vi "AutoTask Controller.vi"(8 "error in":errorcluster) -> ()   [LabVIEW 2016]
doc: "This VI executes continuously carrying out the current operation and responding to updates or new operations. It will often contain the timing or control code that is difficult to place directly in TeleOp. This VI generally opens all sensors and motors and isolates the rest of the robot code from knowing how the operations are carried out."
uses:
  AutoTask Setpoints.ctl
  AutoTask Operations.ctl
  <vilib>/Rock Robotics/Network Tables/NT Read Number.vi
  <vilib>/Rock Robotics/Network Tables/NT Write String.vi
  NavX/navX Library v2/navX Library v2.lvlib
  <vilib>/Rock Robotics/Network Tables/NT Write Boolean.vi
panel:
  out "Current\nCmd":string
  # "Tip: It may be helpful to observe inputs and sensor values.\nYou may also want to display tuning or debugging controls."
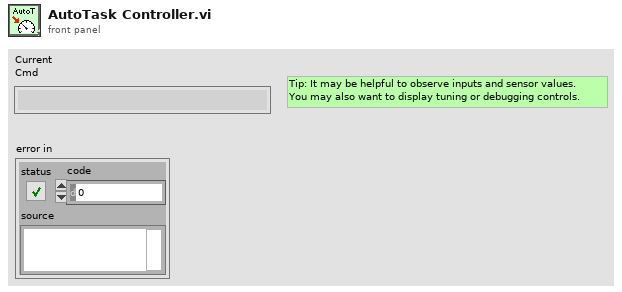
[diagram p1: front panel]
types:
  T1 = typedef "AutoTask Setpoints.ctl" = cluster{"Operation":T2, "Setpoint":dbl, "Duration":dbl, "Speed":dbl, "Angle":dbl, "VDeadband":dbl, "Deadband":dbl}
  T2 = typedef "AutoTask Operations.ctl" = enum16{"Reserve", "Read Current", "Immediate", "DriveDistance", "AutoShoot", "FaceForward", "AutoAlign", "AutoTurn", "DriveToLine", "DriveToIncline", "DriveTillFlat"}
  T3 = typedef "navX Library v2.lvlib/Z900_navX_DeviceTypeDef.ctl" = cluster{"Interface":cluster{"Protocol":T4, "Update Rate (4Hz-60Hz)":u8, "navX Open TypeDef":variant}, "Notify Packet":refnum<notifier>, "Loop VI Refnum":refnum<vi>, "Ready to Close Occurrence Refnum":refnum<k4>}
  T4 = typedef "navX Library v2.lvlib/Z900_navX_ProtocolTypeDef.ctl" = enum16{"SERIAL", "I2C", "SPI"}
  T5 = typedef "Command Status Info.ctl" = cluster{"Name":string, "Status":T6, "notifier out":T7}
  T6 = typedef "Completion Status.ctl" = enum16{"Successful", "Aborted", "Incomplete"}
  T7 = typedef "Completion Notifier.ctl" = refnum<notifier>
  T8 = cluster{"Default Command":T1, "Command Timing":cluster{"Start Time (ms)":u32, "Iterations":i32}, "Command Arguments":cluster{"Command Info":T5, "Description":string, "Default Command":T1, "notifier out":refnum<notifier>, "Subsystem Name":string}}
  T9 = typedef "WPI_EncoderDevRef.ctl" = cluster{"DevStatus":errorcluster, "EncoderIndex":T10, "CounterIndex":T11, "DistancePerCount":dbl, "Decoding Type":T12}
  T10 = typedef "FPGA_EncoderIdx.ctl" = enum8{"Enc 0", "Enc 1", "Enc 2", "Enc 3", "Enc 4", "Enc 5", "Enc 6", "Enc 7", "Invalid"}
  T11 = typedef "FPGA_CounterCtrSystemIndex.ctl" = enum8{"Ctr 0", "Ctr 1", "Ctr 2", "Ctr 3", "Ctr 4", "Ctr 5", "Ctr 6", "Ctr 7", "Invalid"}
  T12 = typedef "WPI_EncoderType.ctl" = enum16{"1x", "2x", "4x"}
  T13 = cluster{"Yaw":dbl, "Roll":dbl, "Pitch":dbl, "Heading":dbl, "Fused Heading":dbl}
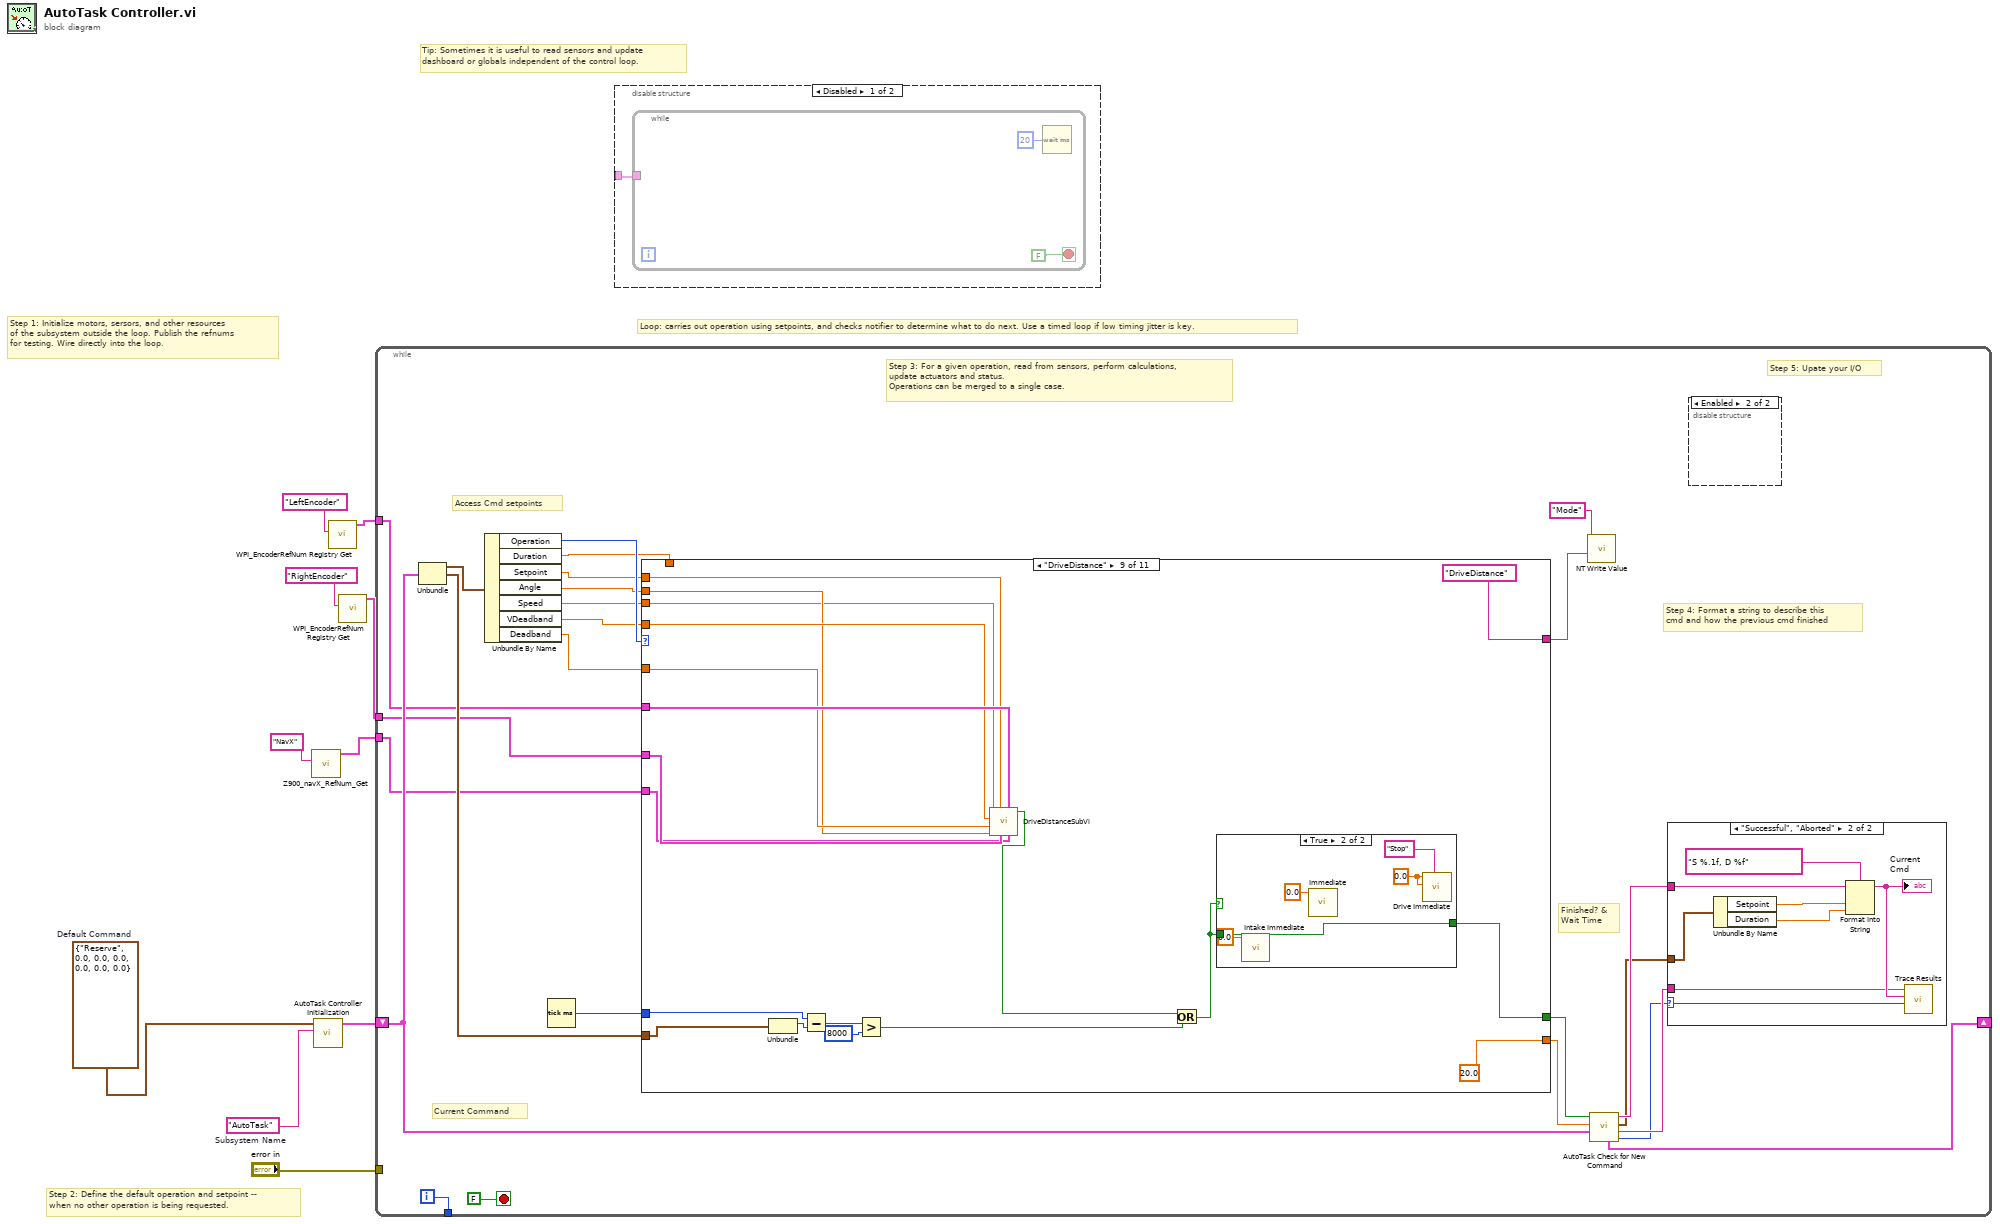
[diagram p0: block diagram]
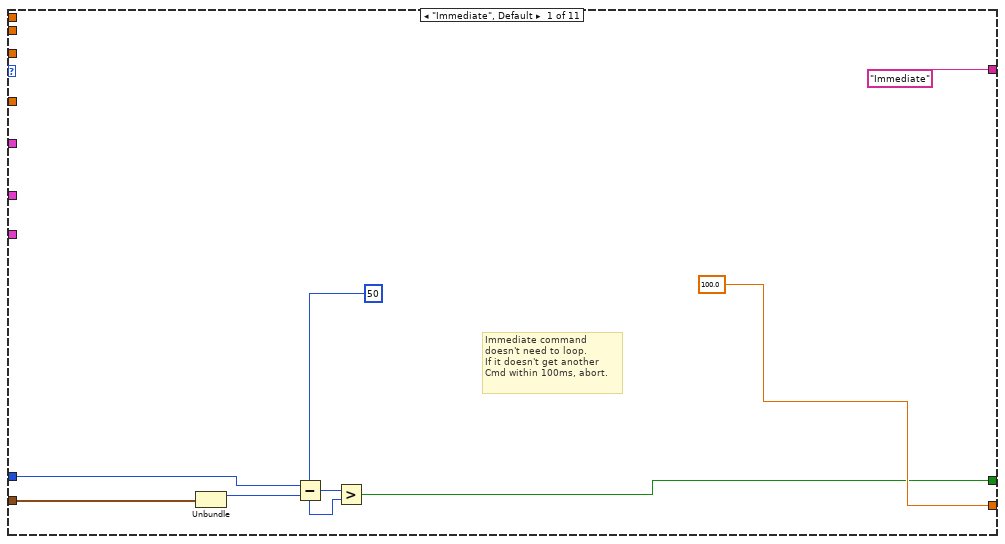
[diagram p3: hidden frame]
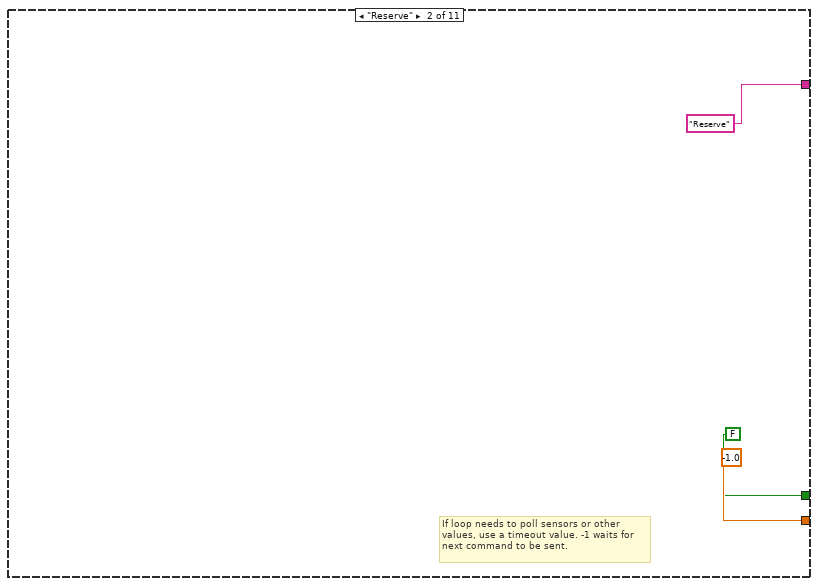
[diagram p4: hidden frame]
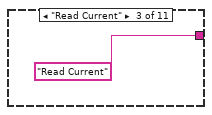
[diagram p5: hidden frame]
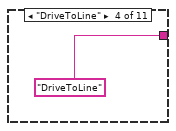
[diagram p6: hidden frame]
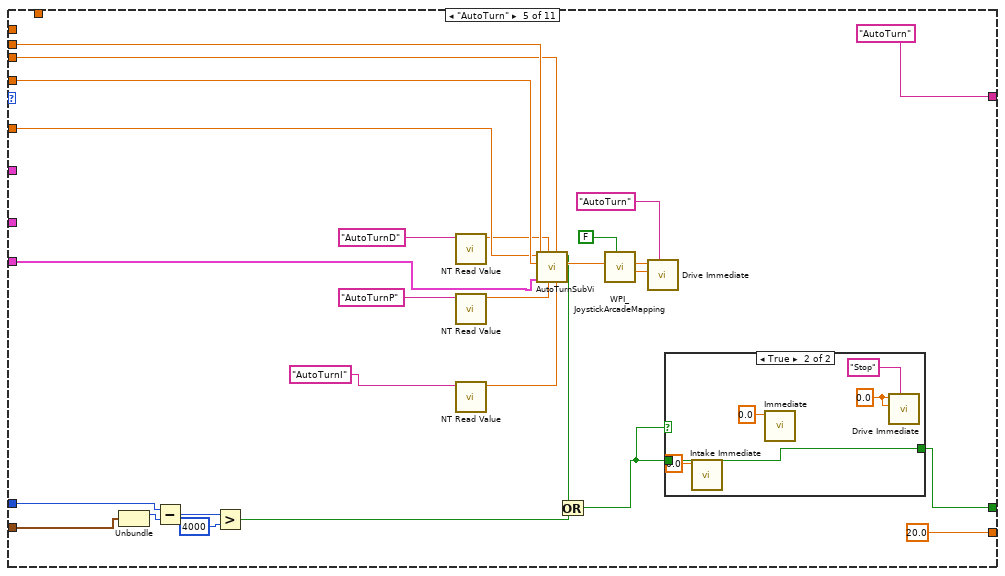
[diagram p7: hidden frame]
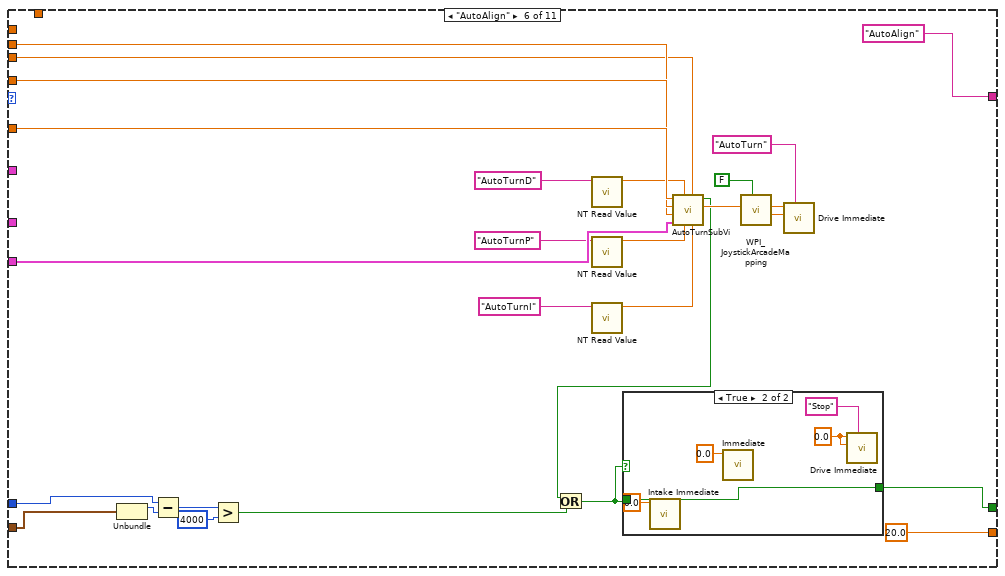
[diagram p9: hidden frame]
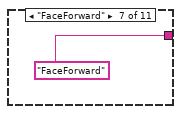
[diagram p11: hidden frame]
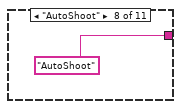
[diagram p12: hidden frame]
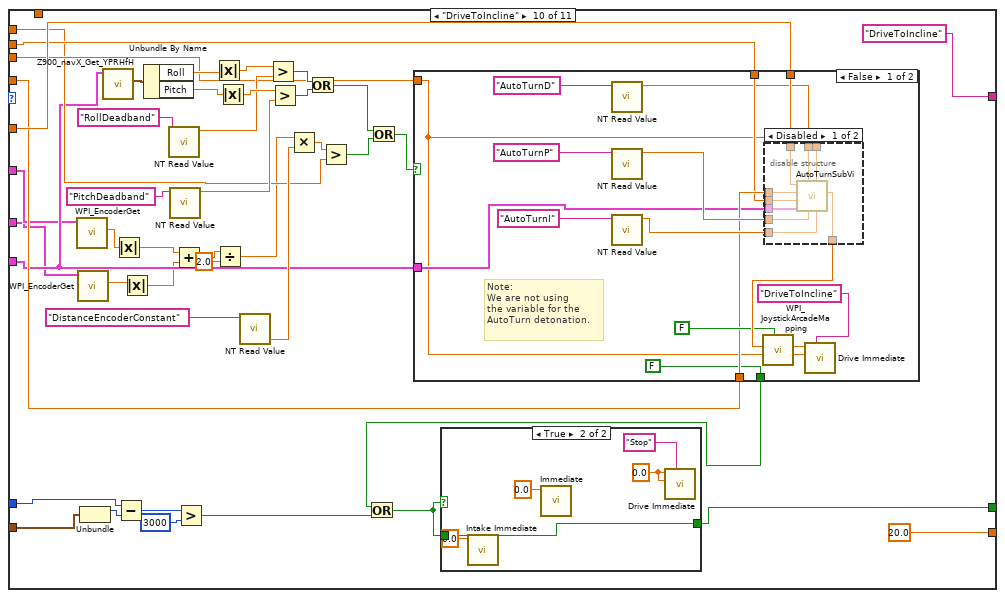
[diagram p14: hidden frame]
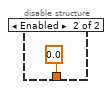
[diagram p16: hidden frame]
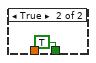
[diagram p17: hidden frame]
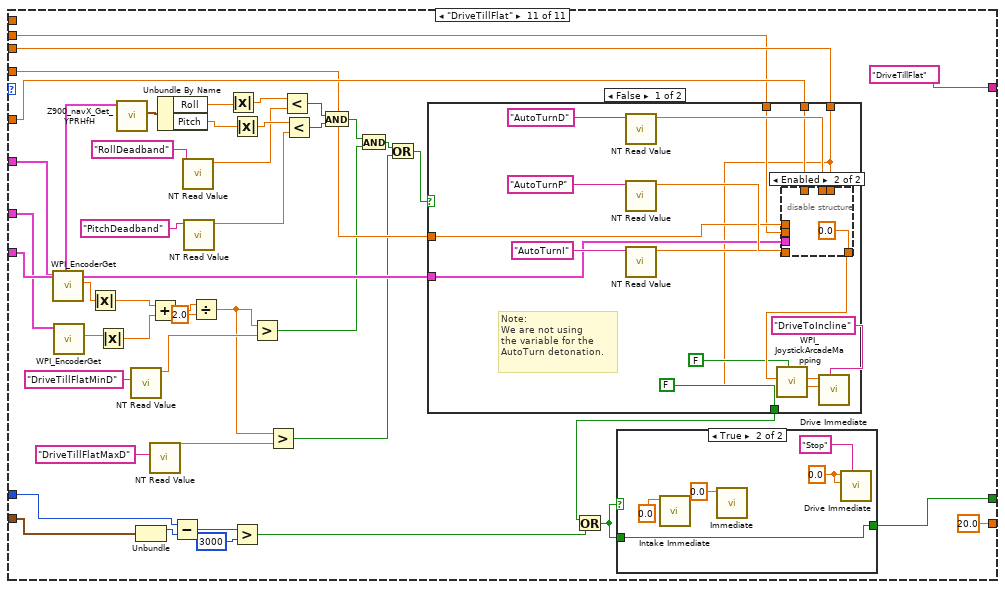
[diagram p18: hidden frame]
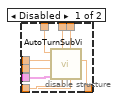
[diagram p20: hidden frame]
diagram:
  w7 = T1 {"Operation"=enum."Reserve", "Setpoint"=0.0, "Duration"=0.0, "Speed"=0.0, "Angle"=0.0, "VDeadband"=0.0, "Deadband"=0.0}  # Default Command
  w8 = "AutoTask"  # Subsystem Name
  # "Tip: Sometimes it is useful to read sensors and update\ndashboard or globals independent of the control loop."
  # "Step 2: Define the default operation and setpoint --\nwhen no other operation is being requested."
  # "Step 1: Initialize motors, sersors, and other resources\nof the subsystem outside the loop. Publish the refnums\nfor testing. Wire directly into the loop."
  # "Loop: carries out operation using setpoints, and checks notifier to determine what to do next. Use a timed loop if low timing jitter is key."
  n1 = call "Z900_navX_RefNum_Get.vi"("refnum name"="NavX") -> ("navX Device"=w6:T3)  [unwired: 9 in, 1 out]
  n2 = call "AutoTask Controller Initialization.vi"("Subsystem Name"=w8, "Default Command"=w7) -> ("Command Info"=w9:T8)  [unwired: 9 in]
  n3 = call <vilib>:"WPI_EncoderRefNum Registry Get.vi"("refnum name"="LeftEncoder") -> ("EncoderDevRef"=w2:T9)  [unwired: 9 in, 1 out]
  n4 = call <vilib>:"WPI_EncoderRefNum Registry Get.vi"("refnum name"="RightEncoder") -> ("EncoderDevRef"=w1:T9)  [unwired: 9 in, 1 out]
  n5 = while {
    shift-right: [w26] -> _
    shift-left: w9 -> [w27]
    tunnel: [w34] -> _
    tunnel: "error in" -> [_]
    tunnel: w6 -> [w19]
    tunnel: w2 -> [w15]
    tunnel: w1 -> [w14]
    i -> [w34]
    stop <- FALSE stop-if-true
    # "Step 5: Upate your I/O"
    # "Step 4: Format a string to describe this\ncmd and how the previous cmd finished"
    # "Current Command"
    # "Access Cmd setpoints"
    # "Finished? &\nWait Time"
    # "Step 3: For a given operation, read from sensors, perform calculations,\nupdate actuators and status.\nOperations can be merged to a single case."
    n6 = Unbundle(w27) -> ("Default Command"=w33:T1, "Command Timing"=w29:cluster{"Start Time (ms)":u32, "Iterations":i32})  [unwired: 1 out]
    n7 = Unbundle By Name(w33) -> ("Operation"=w32:T2, "Duration"=w31:dbl, "Setpoint"=w28:dbl, "Angle"=w18:dbl, "Speed"=w11:dbl, "VDeadband"=w13:dbl, "Deadband"=w12:dbl)
    n8 = Tick Count (ms)() -> (millisecond timer value=w30:u32)
    n9 = case shown="\"DriveDistance\"" w32 {
      tunnel: [100.0 -1.0 _ _ 20.0 20.0 _ _ 20.0 20.0 20.0] -> w24
      tunnel: [w37 FALSE ("ignore previous (F)") _ _ w56 w90 _ _ w125 w150 w227] -> w25
      tunnel: w29 -> [w39 _ _ _ w52 w84 _ _ w119 w144 w221]
      tunnel: w31 -> [_ _ _ _ _ _ _ _ _ _ _]
      tunnel: w30 -> [w38 _ _ _ w51 w85 _ _ w120 w145 w222]
      tunnel: w28 -> [_ _ _ _ _ _ _ _ w132 w164 _]
      tunnel: w19 -> [_ _ _ _ w73 w103 _ _ w126 w160 w247]
      tunnel: w18 -> [_ _ _ _ w74 w105 _ _ w129 w171 w249]
      tunnel: ["Immediate" "Reserve" "Read Current" "DriveToLine" "AutoTurn" "AutoAlign" "FaceForward" "AutoShoot" "DriveDistance" "DriveToIncline" "DriveTillFlat"] -> w16
      tunnel: w13 -> [_ _ _ _ w71 w106 _ _ w131 w172 w250]
      tunnel: w12 -> [_ _ _ _ w70 w107 _ _ w130 w173 w251]
      tunnel: w15 -> [_ _ _ _ _ _ _ _ w134 w159 w237]
      tunnel: w14 -> [_ _ _ _ _ _ _ _ w133 w158 w236]
      tunnel: w11 -> [_ _ _ _ w58 w91 _ _ w127 w170 w252]
      frame "Immediate", Default {
        # "Immediate command\ndoesn't need to loop.\nIf it doesn't get another\nCmd within 100ms, abort."
        n10 = Unbundle(w39) -> ("Start Time (ms)"=w42:u32)  [unwired: 1 out]
        n11 = Subtract(x=w38, y=w42) -> (x-y=w41:u32)
        n12 = Greater?(x=w41, y=u8 50 ("Left Motor")) -> (0:w37:bool)
      }
      frame "Reserve" {
        # "If loop needs to poll sensors or other\nvalues, use a timeout value. -1 waits for\nnext command to be sent."
      }
      frame "Read Current" {
      }
      frame "DriveToLine" {
      }
      frame "AutoTurn" {
        n13 = Unbundle(w52) -> ("Start Time (ms)"=w55:u32)  [unwired: 1 out]
        n14 = Subtract(x=w51, y=w55) -> (x-y=w54:u32)
        n15 = Greater?(x=w54, y=u32 4000 ("Left Motor")) -> (0:w49:bool)
        n16 = call-poly <vilib>:"NT Read Value.vi"("Name"="AutoTurnD") -> ("Numeric"=w60:dbl)  [unwired: 9 in, 1 out]
        n17 = call-poly <vilib>:"NT Read Value.vi"("Name"="AutoTurnP") -> ("Numeric"=w59:dbl)  [unwired: 9 in, 1 out]
        n18 = call-poly <vilib>:"NT Read Value.vi"("Name"="AutoTurnI") -> ("Numeric"=w61:dbl)  [unwired: 9 in, 1 out]
        n19 = call "AutoTurnSubVi.vi"("I"=w61, "Speed"=w58, "P"=w59, "D"=w60, "navX Device"=w73, "Angle"=w74, "VDeadband"=w71, "Deadband"=w70) -> ("Output"=w66:dbl, "Boolean"=w57:bool)  [unwired: 2 in]
        n20 = Or(x=w57, y=w49) -> (x .or. y?=w50:bool)
        n21 = call <vilib>:"WPI_JoystickArcadeMapping.vi"("Square Inputs"=FALSE, "X axis value"=w66) -> ("Right Motor Value"=w68:dbl, "Left Motor Value"=w67:dbl)  [unwired: 8 in]
        n22 = call "Drive Immediate.vi"("Description"="AutoTurn", "Right Setpoint"=w68, "Left Setpoint"=w67) -> ()  [unwired: 8 in, 1 out]
        n23 = case shown="True" w50 {
          tunnel: [w76 w81] -> w56
          tunnel: w50 -> [w76 w81]
          frame False {
          }
          frame True {
            w79 = 0.0
            n24 = call "Intake Immediate.vi"("Setpoint"=0.0) -> ()  [unwired: 10 in, 1 out]
            n25 = call "Immediate.vi"("Setpoint"=0.0) -> ()  [unwired: 10 in, 1 out]
            n26 = call "Drive Immediate.vi"("Description"="Stop", "Right Setpoint"=w79, "Left Setpoint"=w79) -> ()  [unwired: 8 in, 1 out]
          }
        }
      }
      frame "AutoAlign" {
        n27 = Unbundle(w84) -> ("Start Time (ms)"=w89:u32)  [unwired: 1 out]
        n28 = Subtract(x=w85, y=w89) -> (x-y=w88:u32)
        n29 = Greater?(x=w88, y=u32 4000 ("Left Motor")) -> (0:w86:bool)
        n30 = call-poly <vilib>:"NT Read Value.vi"("Name"="AutoTurnD") -> ("Numeric"=w92:dbl)  [unwired: 9 in, 1 out]
        n31 = call-poly <vilib>:"NT Read Value.vi"("Name"="AutoTurnP") -> ("Numeric"=w94:dbl)  [unwired: 9 in, 1 out]
        n32 = call-poly <vilib>:"NT Read Value.vi"("Name"="AutoTurnI") -> ("Numeric"=w93:dbl)  [unwired: 9 in, 1 out]
        n33 = call "AutoTurnSubVi.vi"("I"=w93, "Speed"=w91, "P"=w94, "D"=w92, "navX Device"=w103, "Angle"=w105, "VDeadband"=w106, "Deadband"=w107) -> ("Output"=w98:dbl, "Boolean"=w83:bool)  [unwired: 2 in]
        n34 = Or(x=w83, y=w86) -> (x .or. y?=w82:bool)
        n35 = case shown="True" w82 {
          tunnel: [w109 w114] -> w90
          tunnel: w82 -> [w109 w114]
          frame False {
          }
          frame True {
            w112 = 0.0
            n36 = call "Intake Immediate.vi"("Setpoint"=0.0) -> ()  [unwired: 10 in, 1 out]
            n37 = call "Immediate.vi"("Setpoint"=0.0) -> ()  [unwired: 10 in, 1 out]
            n38 = call "Drive Immediate.vi"("Description"="Stop", "Right Setpoint"=w112, "Left Setpoint"=w112) -> ()  [unwired: 8 in, 1 out]
          }
        }
        n39 = call <vilib>:"WPI_JoystickArcadeMapping.vi"("Square Inputs"=FALSE, "X axis value"=w98) -> ("Right Motor Value"=w101:dbl, "Left Motor Value"=w100:dbl)  [unwired: 8 in]
        n40 = call "Drive Immediate.vi"("Description"="AutoTurn", "Right Setpoint"=w101, "Left Setpoint"=w100) -> ()  [unwired: 8 in, 1 out]
      }
      frame "FaceForward" {
      }
      frame "AutoShoot" {
      }
      frame "DriveDistance" {
        n41 = Unbundle(w119) -> ("Start Time (ms)"=w124:u32)  [unwired: 1 out]
        n42 = Subtract(x=w120, y=w124) -> (x-y=w123:u32)
        n43 = Greater?(x=w123, y=u32 8000 ("Left Motor")) -> (0:w121:bool)
        n44 = call "DriveDistanceSubVi.vi"("navX Device"=w126, "EncoderDevRefLeft"=w134, "EncoderDevRefRight"=w133, "Setpoint"=w132, "Angle"=w129, "Deadband"=w130, "VDeadband"=w131, "Speed"=w127) -> ("Boolean"=w118:bool)  [unwired: 3 in]
        n45 = Or(x=w118, y=w121) -> (x .or. y?=w117:bool)
        n46 = case shown="True" w117 {
          tunnel: [w136 w141] -> w125
          tunnel: w117 -> [w136 w141]
          frame False {
          }
          frame True {
            w139 = 0.0
            n47 = call "Intake Immediate.vi"("Setpoint"=0.0) -> ()  [unwired: 10 in, 1 out]
            n48 = call "Immediate.vi"("Setpoint"=0.0) -> ()  [unwired: 10 in, 1 out]
            n49 = call "Drive Immediate.vi"("Description"="Stop", "Right Setpoint"=w139, "Left Setpoint"=w139) -> ()  [unwired: 8 in, 1 out]
          }
        }
      }
      frame "DriveToIncline" {
        n50 = call <vilib>:"WPI_EncoderGet.vi"("EncoderDevRef"=w159) -> ("Distance"=w156:dbl)  [unwired: 5 in, 5 out]
        n51 = call <vilib>:"WPI_EncoderGet.vi"("EncoderDevRef"=w158) -> ("Distance"=w157:dbl)  [unwired: 5 in, 5 out]
        n52 = Unbundle(w144) -> ("Start Time (ms)"=w149:u32)  [unwired: 1 out]
        n53 = call "Z900_navX_Get_YPRHfH.vi"("navX Device"=w160) -> ("YRPHfH"=w184:T13)  [unwired: 7 in, 3 out]
        n54 = Absolute Value(x=w156) -> (abs(x)=w155:dbl)
        n55 = Subtract(x=w145, y=w149) -> (x-y=w148:u32)
        n56 = Absolute Value(x=w157) -> (abs(x)=w154:dbl)
        n57 = Unbundle By Name(w184) -> ("Roll"=w183:dbl, "Pitch"=w180:dbl)
        n58 = call-poly <vilib>:"NT Read Value.vi"("Name"="RollDeadband") -> ("Numeric"=w177:dbl)  [unwired: 9 in, 1 out]
        n59 = call-poly <vilib>:"NT Read Value.vi"("Name"="PitchDeadband") -> ("Numeric"=w176:dbl)  [unwired: 9 in, 1 out]
        n60 = Add(x=w155, y=w154) -> (x+y=w153:dbl)
        n61 = Greater?(x=w148, y=u32 3000 ("Left Motor")) -> (0:w146:bool)
        n62 = Absolute Value(x=w183) -> (abs(x)=w182:dbl)
        n63 = Divide(x=w153, y=2.0) -> (x/y=w151:dbl)
        n64 = Absolute Value(x=w180) -> (abs(x)=w181:dbl)
        n65 = call-poly <vilib>:"NT Read Value.vi"("Name"="DistanceEncoderConstant") -> ("Numeric"=w166:dbl)  [unwired: 9 in, 1 out]
        n66 = Greater?(x=w182, y=w177) -> (0:w174:bool)
        n67 = Greater?(x=w181, y=w176) -> (0:w175:bool)
        n68 = Multiply(x=w151, y=w166) -> (x*y=w165:dbl)
        n69 = Or(x=w174, y=w175) -> (x .or. y?=w163:bool)
        n70 = Greater?(x=w165, y=w164) -> (0:w162:bool)
        n71 = Or(x=w163, y=w162) -> (x .or. y?=w161:bool)
        n72 = case shown="False" w161 {
          tunnel: w173 -> [w197 _]
          tunnel: w172 -> [w196 _]
          tunnel: w171 -> [w195 _]
          tunnel: w170 -> [w193 _]
          tunnel: w160 -> [w194 _]
          tunnel: [FALSE TRUE] -> w143
          frame False {
            # "Note:\nWe are not using\nthe variable for the\nAutoTurn detonation."
            n73 = call-poly <vilib>:"NT Read Value.vi"("Name"="AutoTurnD") -> ("Numeric"=w191:dbl)  [unwired: 9 in, 1 out]
            n74 = call-poly <vilib>:"NT Read Value.vi"("Name"="AutoTurnP") -> ("Numeric"=w206:dbl)  [unwired: 9 in, 1 out]
            n75 = call-poly <vilib>:"NT Read Value.vi"("Name"="AutoTurnI") -> ("Numeric"=w205:dbl)  [unwired: 9 in, 1 out]
            n76 = disable-structure shown="Disabled" {
              disable-tunnel: [w216 0.0 ("X axis value")] -> w207
              disable-tunnel: w206 -> [w215 _]
              disable-tunnel: w205 -> [w214 _]
              disable-tunnel: w197 -> [w213 _]
              disable-tunnel: w196 -> [w212 _]
              disable-tunnel: w195 -> [w211 _]
              disable-tunnel: w194 -> [w210 _]
              disable-tunnel: w193 -> [w209 _]
              disable-tunnel: w191 -> [w208 _]
              frame Disabled {
                n77 = call "AutoTurnSubVi.vi"("I"=w214, "Speed"=w209, "P"=w215, "D"=w208, "navX Device"=w210, "Angle"=w211, "VDeadband"=w212, "Deadband"=w213) -> ("Output"=w216:dbl)  [unwired: 2 in, 1 out]
              }
              frame Enabled {
              }
            }
            n78 = call <vilib>:"WPI_JoystickArcadeMapping.vi"("Square Inputs"=FALSE, "Y axis value"=w193, "X axis value"=w207) -> ("Right Motor Value"=w199:dbl, "Left Motor Value"=w198:dbl)  [unwired: 7 in]
            n79 = call "Drive Immediate.vi"("Description"="DriveToIncline", "Right Setpoint"=w199, "Left Setpoint"=w198) -> ()  [unwired: 8 in, 1 out]
          }
          frame True {
          }
        }
        n80 = Or(x=w143, y=w146) -> (x .or. y?=w142:bool)
        n81 = case shown="True" w142 {
          tunnel: [w185 w190] -> w150
          tunnel: w142 -> [w185 w190]
          frame False {
          }
          frame True {
            w188 = 0.0
            n82 = call "Intake Immediate.vi"("Setpoint"=0.0) -> ()  [unwired: 10 in, 1 out]
            n83 = call "Immediate.vi"("Setpoint"=0.0) -> ()  [unwired: 10 in, 1 out]
            n84 = call "Drive Immediate.vi"("Description"="Stop", "Right Setpoint"=w188, "Left Setpoint"=w188) -> ()  [unwired: 8 in, 1 out]
          }
        }
      }
      frame "DriveTillFlat" {
        n85 = call <vilib>:"WPI_EncoderGet.vi"("EncoderDevRef"=w237) -> ("Distance"=w238:dbl)  [unwired: 5 in, 5 out]
        n86 = call <vilib>:"WPI_EncoderGet.vi"("EncoderDevRef"=w236) -> ("Distance"=w243:dbl)  [unwired: 5 in, 5 out]
        n87 = Absolute Value(x=w238) -> (abs(x)=w242:dbl)
        n88 = Absolute Value(x=w243) -> (abs(x)=w241:dbl)
        n89 = call "Z900_navX_Get_YPRHfH.vi"("navX Device"=w247) -> ("YRPHfH"=w263:T13)  [unwired: 7 in, 3 out]
        n90 = call-poly <vilib>:"NT Read Value.vi"("Name"="DriveTillFlatMinD") -> ("Numeric"=w233:dbl)  [unwired: 9 in, 1 out]
        n91 = Unbundle(w221) -> ("Start Time (ms)"=w226:u32)  [unwired: 1 out]
        n92 = Add(x=w242, y=w241) -> (x+y=w240:dbl)
        n93 = call-poly <vilib>:"NT Read Value.vi"("Name"="DriveTillFlatMaxD") -> ("Numeric"=w231:dbl)  [unwired: 9 in, 1 out]
        n94 = Unbundle By Name(w263) -> ("Roll"=w262:dbl, "Pitch"=w259:dbl)
        n95 = Subtract(x=w222, y=w226) -> (x-y=w225:u32)
        n96 = call-poly <vilib>:"NT Read Value.vi"("Name"="RollDeadband") -> ("Numeric"=w256:dbl)  [unwired: 9 in, 1 out]
        n97 = call-poly <vilib>:"NT Read Value.vi"("Name"="PitchDeadband") -> ("Numeric"=w255:dbl)  [unwired: 9 in, 1 out]
        n98 = Divide(x=w240, y=2.0) -> (x/y=w230:dbl)
        n99 = Absolute Value(x=w262) -> (abs(x)=w261:dbl)
        n100 = Absolute Value(x=w259) -> (abs(x)=w260:dbl)
        n101 = Greater?(x=w225, y=u32 3000 ("Left Motor")) -> (0:w223:bool)
        n102 = Greater?(x=w230, y=w233) -> (0:w232:bool)
        n103 = Greater?(x=w230, y=w231) -> (0:w229:bool)
        n104 = Less?(x=w261, y=w256) -> (x < y?=w253:bool)
        n105 = Less?(x=w260, y=w255) -> (x < y?=w254:bool)
        n106 = And(x=w253, y=w254) -> (x .and. y?=w246:bool)
        n107 = And(x=w246, y=w232) -> (x .and. y?=w245:bool)
        n108 = Or(x=w245, y=w229) -> (x .or. y?=w244:bool)
        n109 = case shown="False" w244 {
          tunnel: [FALSE TRUE] -> w220
          tunnel: w252 -> [w270 _]
          tunnel: w251 -> [w275 _]
          tunnel: w250 -> [w274 _]
          tunnel: w249 -> [w273 _]
          tunnel: w247 -> [w271 _]
          frame False {
            # "Note:\nWe are not using\nthe variable for the\nAutoTurn detonation."
            n110 = call-poly <vilib>:"NT Read Value.vi"("Name"="AutoTurnD") -> ("Numeric"=w276:dbl)  [unwired: 9 in, 1 out]
            n111 = call-poly <vilib>:"NT Read Value.vi"("Name"="AutoTurnP") -> ("Numeric"=w285:dbl)  [unwired: 9 in, 1 out]
            n112 = call-poly <vilib>:"NT Read Value.vi"("Name"="AutoTurnI") -> ("Numeric"=w272:dbl)  [unwired: 9 in, 1 out]
            n113 = disable-structure shown="Enabled" {
              disable-tunnel: [w295 0.0 ("X axis value")] -> w286
              disable-tunnel: w285 -> [w294 _]
              disable-tunnel: w276 -> [w293 _]
              disable-tunnel: w270 -> [w292 _]
              disable-tunnel: w275 -> [w291 _]
              disable-tunnel: w274 -> [w290 _]
              disable-tunnel: w273 -> [w289 _]
              disable-tunnel: w272 -> [w288 _]
              disable-tunnel: w271 -> [w287 _]
              frame Disabled {
                n114 = call "AutoTurnSubVi.vi"("I"=w288, "Speed"=w292, "P"=w294, "D"=w293, "navX Device"=w287, "Angle"=w289, "VDeadband"=w290, "Deadband"=w291) -> ("Output"=w295:dbl)  [unwired: 2 in, 1 out]
              }
              frame Enabled {
              }
            }
            n115 = call <vilib>:"WPI_JoystickArcadeMapping.vi"("Square Inputs"=FALSE, "Y axis value"=w270, "X axis value"=w286) -> ("Right Motor Value"=w279:dbl, "Left Motor Value"=w278:dbl)  [unwired: 7 in]
            n116 = call "Drive Immediate.vi"("Description"="DriveToIncline", "Right Setpoint"=w279, "Left Setpoint"=w278) -> ()  [unwired: 8 in, 1 out]
          }
          frame True {
          }
        }
        n117 = Or(x=w220, y=w223) -> (x .or. y?=w219:bool)
        n118 = case shown="True" w219 {
          tunnel: [w264 w265] -> w227
          tunnel: w219 -> [w264 w265]
          frame False {
          }
          frame True {
            w268 = 0.0
            n119 = call "Intake Immediate.vi"("Setpoint"=0.0) -> ()  [unwired: 10 in, 1 out]
            n120 = call "Immediate.vi"("Setpoint"=0.0) -> ()  [unwired: 10 in, 1 out]
            n121 = call "Drive Immediate.vi"("Description"="Stop", "Right Setpoint"=w268, "Left Setpoint"=w268) -> ()  [unwired: 8 in, 1 out]
          }
        }
      }
    }
    n122 = call-poly <vilib>:"NT Write Value.vi"("String"=w16, "Name"="Mode") -> ()  [unwired: 9 in, 1 out]
    n123 = call "AutoTask Check for New Command.vi"("Current Command"=w27, "Wait time (ms)"=w24, "Finished?"=w25) -> ("Completion"=w20:T6, "Subsystem Name"=w21:string, "Current Command"=w22:T1, "Initial Trace String"=w23:string, "NextCommand"=w26:T8)  [unwired: 4 in]
    n124 = case shown="\"Successful\", \"Aborted\"" w20 {
      selector: w20 -> [_ w305]
      tunnel: w23 -> [_ w301]
      tunnel: w22 -> [_ w302]
      tunnel: w21 -> [_ w298]
      frame "Incomplete", Default {
        # "Continuing current command"
      }
      frame "Successful", "Aborted" {
        # "Report and setup for next command"
        n125 = Unbundle By Name(w302) -> ("Setpoint"=w304:dbl, "Duration"=w299:dbl)
        n126 = Format Into String(format string="S %.1f, D %f", initial string=w301, w304, w299) -> (resulting string=w300:string)  [unwired: 1 in, 1 out]
        "Current\nCmd" <- w300
        n127 = call <vilib>:"Trace Results.vi"("Status of previous command"=w305, "Description"=w300, "Subsystem"=w298) -> ()  [unwired: 9 in]
      }
    }
    n128 = disable-structure shown="Enabled" {
      frame Disabled {
        # "Publish"
        n129 = call-poly <vilib>:"NT Write Value.vi"() -> ()  [unwired: 11 in, 1 out]
      }
      frame Enabled {
      }
    }
  }
  n130 = disable-structure shown="Disabled" {
    disable-tunnel: _ -> [w306 _]
    frame Disabled {
      n131 = while {
        tunnel: w306 -> [_]
        stop <- FALSE stop-if-true
        n132 = Wait (ms)(milliseconds to wait=u32 20) -> ()  [unwired: 1 out]
      }
    }
    frame Enabled {
    }
  }
